vi "Close.vi"(8 "error in (no error)":errorcluster, 11 "ASIA Pump C":T1 {"channel" min=0 max=1 step=1}) -> (0 "error out":errorcluster, 2 "Task Completed":bool, 3 "ASIA Pump C":T1 {"channel" min=0 max=1 step=1})   [LabVIEW 2018, in "ASIA Pump.lvlib"]
uses:
  ASIA Pump.lvlib
  Pump Settings.ctl
  Program Files (x86)/Pfizer/FAST/data/AsiaPumpInterface.dll
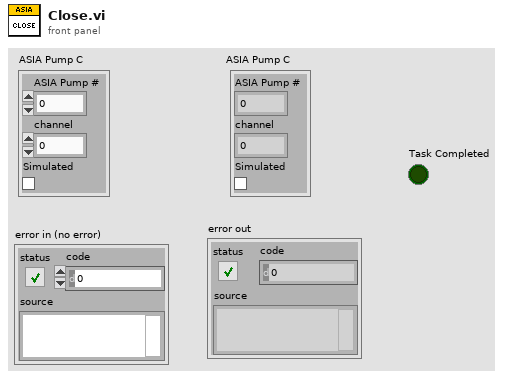
[diagram p1: front panel]
types:
  T1 = typedef "ASIA Pump.lvlib/Pump Settings.ctl" = cluster{"ASIA Pump #":i32, "channel":i32, "Simulated":bool}
  T2 = cluster{"Busy":bool, "PumpCnt":dbl, "RemoteEntered":bool, "OverpressureSet":bool}[]
  T3 = cluster{"Busy":bool, "PumpCnt":dbl, "RemoteEntered":bool, "OverpressureSet":bool}
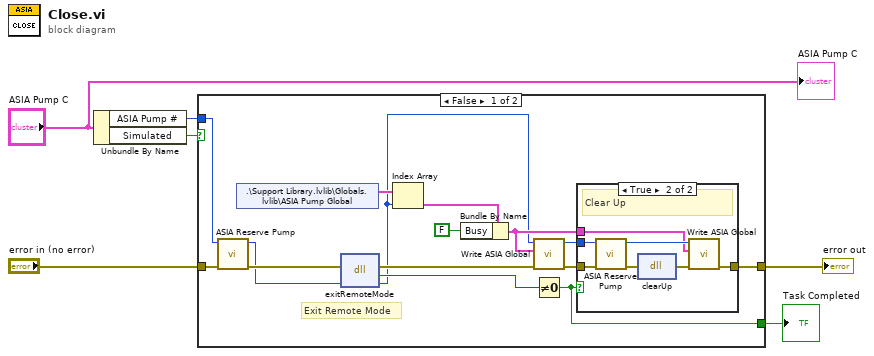
[diagram p0: block diagram]
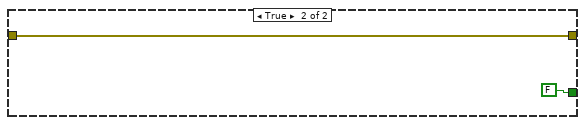
[diagram p3: hidden frame]
diagram:
  n1 = Unbundle By Name("ASIA Pump C") -> ("ASIA Pump #"=w2:i32, "Simulated"=w1:bool)
  n2 = case shown="False" w1 {
    tunnel: "error in (no error)" -> [w18 w31]
    tunnel: w2 -> [w16 _]
    tunnel: [w21 w31] -> w4
    tunnel: [w19 FALSE] -> w3
    frame False {
      # "Exit Remote Mode"
      n3 = call "ASIA Reserve Pump.vi"("error in (no error)"=w18, "ASIA Pump #"=w16) -> ("error out"=w17:errorcluster, "ASIA Pump #"=w15:i32)  [unwired: 8 in]
      n4 = shared-variable ".\\Support Library.lvlib\\Globals.lvlib\\ASIA Pump Global"() -> (w9:T2)  [unwired: 1 in, 1 out]
      n5 = dll-call lib="C:/Program Files (x86)/Pfizer/FAST/data/AsiaPumpInterface.dll" fn="exitRemoteMode"(error in=w17, "pumpNum"=w15) -> (error out=w14:errorcluster, "Bool"=w20:u8, "pumpNum"=w8:u32)  [unwired: 2 in, 1 out]
      n6 = Index Array(array=w9, index=w8) -> (element=w7:T3)
      n7 = Bundle By Name(cluster=w7, "Busy"=FALSE) -> (w10:T3)
      n8 = call "Write ASIA Global.vi"("error in (no error)"=w14, "ASIA Global"=w10, "Pump Number"=w8) -> ("error out"=w13:errorcluster, "Pump Number"=w12:i32)  [unwired: 7 in]
      n9 = Not Equal To 0?(x=w20) -> (x != 0?=w19:bool)
      n10 = case shown="True" w19 {
        tunnel: w13 -> [w22 w29]
        tunnel: [w22 w26] -> w21
        tunnel: w12 -> [_ w25]
        tunnel: w10 -> [_ w23]
        frame False {
          # "Error"
        }
        frame True {
          # "Clear Up"
          n11 = call "ASIA Reserve Pump.vi"("error in (no error)"=w29, "ASIA Pump #"=w25) -> ("error out"=w28:errorcluster, "ASIA Pump #"=w24:i32)  [unwired: 8 in]
          n12 = dll-call lib="C:/Program Files (x86)/Pfizer/FAST/data/AsiaPumpInterface.dll" fn="clearUp"(error in=w28) -> (error out=w27:errorcluster)  [unwired: 3 in, 1 out]
          n13 = call "Write ASIA Global.vi"("error in (no error)"=w27, "ASIA Global"=w23, "Pump Number"=w24) -> ("error out"=w26:errorcluster)  [unwired: 7 in, 1 out]
        }
      }
    }
    frame True {
    }
  }
  "error out" <- w4
  "Task Completed" <- w3
  "ASIA Pump C" <- "ASIA Pump C"
